vi "Strain_max.vi"(8 "error in (no error)":errorcluster caption="err in", 11 "Q_data":T1) -> (0 "error out":errorcluster caption="err out", 3 "Max Strain":dbl)   [LabVIEW 2016]
uses:
  Ctrls/raw Q data.ctl
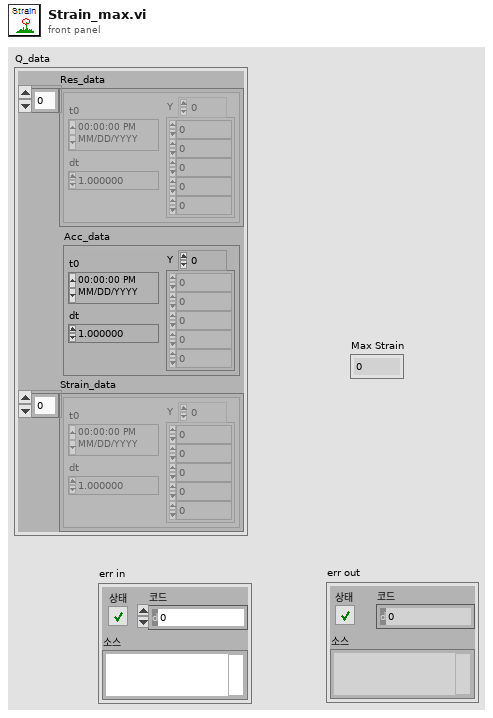
[diagram p1: front panel]
types:
  T1 = typedef "raw Q data.ctl" = cluster{"Res_data":waveform(dbl)[], "Acc_data":waveform(dbl), "Strain_data":waveform(dbl)[]}
  T2 = typedef "Total data.ctl" = cluster{"Raw Data":T1, "Resister result data":T3, "Result Table update":cluster{"Num":u32[], "Resister 1~5":u8[][], "Resister 6~10":u8[][], "Resister 11~15":u8[][]}, "Strain Data":cluster{"Strain 1":dbl, "Strain 2":dbl, "Strain 3":dbl, "Strain 4":dbl}, "Acc Result":cluster{"Acc Peak":dbl, "Acc time":dbl, "Acc area":dbl}, "STATUS":cluster{"status":string, "all_fail":bool, "emg":bool, "cycle":u16, "file name":string}, "Speed":dbl, "Acc peak time":dbl, "Max Strain":dbl, "Resistor at peak":cluster{"[0]":dbl, "[1]":dbl, "[2]":dbl, "[3]":dbl, "[4]":dbl, "[5]":dbl, "[6]":dbl, "[7]":dbl, "[8]":dbl, "[9]":dbl, "[10]":dbl, "[11]":dbl, "[12]":dbl, "[13]":dbl, "[14]":dbl}, "Acc peak index":u32, "time":string, "Cycle finish":bool, "Resistor at ini":cluster{"[0]":dbl, "[1]":dbl, "[2]":dbl, "[3]":dbl, "[4]":dbl, "[5]":dbl, "[6]":dbl, "[7]":dbl, "[8]":dbl, "[9]":dbl, "[10]":dbl, "[11]":dbl, "[12]":dbl, "[13]":dbl, "[14]":dbl}}
  T3 = typedef "raw data type.ctl" = cluster{"Resistor values":cluster{"[0]":dbl, "[1]":dbl, "[2]":dbl, "[3]":dbl, "[4]":dbl, "[5]":dbl, "[6]":dbl, "[7]":dbl, "[8]":dbl, "[9]":dbl, "[10]":dbl, "[11]":dbl, "[12]":dbl, "[13]":dbl, "[14]":dbl}, "Resistor tables":u8[], "Pass Fails":bool[]}
  T4 = cluster{"[0]":dbl, "[1]":dbl, "[2]":dbl, "[3]":dbl}
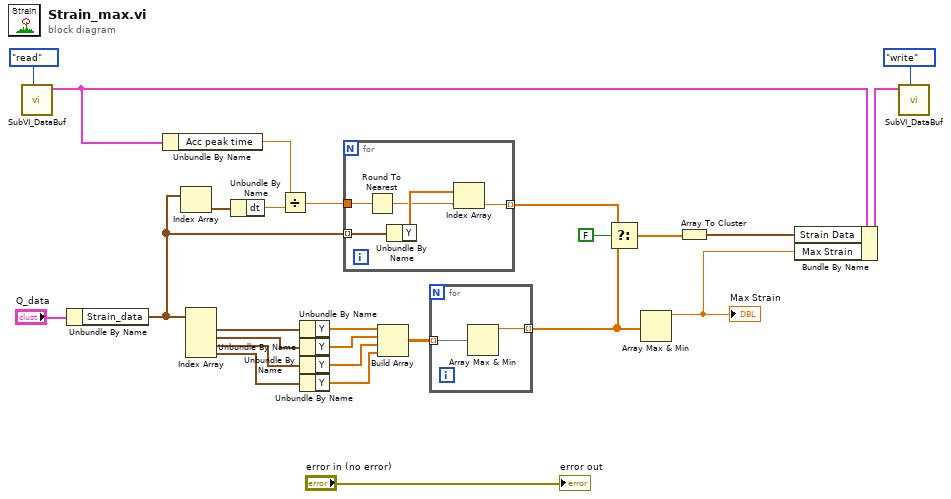
[diagram p0: block diagram]
diagram:
  n1 = call "SubVI_DataBuf.vi"("cmd"=enum16{"ini", "write", "read"}."read") -> ("Total data 2"=w12:T2)  [unwired: 9 in, 1 out]
  n2 = Unbundle By Name("Q_data") -> ("Strain_data"=w11:waveform(dbl)[])
  n3 = Unbundle By Name(w12) -> ("Acc peak time"=w8:dbl)
  n4 = Index Array(array=w11) -> (element=w10:waveform(dbl))  [unwired: 1 in]
  n5 = Index Array(array=w11) -> (element #1=w21:waveform(dbl), element #2=w20:waveform(dbl), element #3=w19:waveform(dbl), element #4=w18:waveform(dbl))  [unwired: 4 in]
  n6 = Unbundle By Name(w10) -> ("dt"=w9:dbl)
  n7 = Divide(x=w8, y=w9) -> (x/y=w7:dbl)
  n8 = Unbundle By Name(w21) -> ("Y"=w17:dbl[])
  n9 = Unbundle By Name(w20) -> ("Y"=w16:dbl[])
  n10 = Unbundle By Name(w19) -> ("Y"=w15:dbl[])
  n11 = Unbundle By Name(w18) -> ("Y"=w14:dbl[])
  n12 = for {
    tunnel: w11 -> [w31] mode=indexing
    tunnel: w7 -> [w30]
    tunnel: [w27] -> w6 mode=indexing
    n13 = Round To Nearest(number=w30) -> (nearest integer value=w28:dbl)
    n14 = Unbundle By Name(w31) -> ("Y"=w29:dbl[])
    n15 = Index Array(array=w29, index=w28) -> (element=w27:dbl)
  }
  n16 = Build Array(w17, w16, w15, w14) -> (w13:dbl[][])
  n17 = for {
    tunnel: w13 -> [w33] mode=indexing
    tunnel: [w32] -> w5 mode=indexing
    n18 = Array Max & Min(array=w33) -> (max value=w32:dbl)  [unwired: 3 out]
  }
  n19 = Select(t=w6, s=FALSE, f=w5) -> (s? t:f=w4:dbl[])
  n20 = Array Max & Min(array=w5) -> (max value=w1:dbl)  [unwired: 3 out]
  "Max Strain" <- w1
  n21 = Array To Cluster(array=w4) -> (cluster=w3:T4)
  n22 = Bundle By Name(cluster=w12, "Strain Data"=w3, "Max Strain"=w1) -> (w23:T2)
  n23 = call "SubVI_DataBuf.vi"("cmd"=enum16{"ini", "write", "read"}."write", "Total data"=w23) -> ()  [unwired: 8 in, 2 out]
  "error out" <- "error in (no error)"
